vi "Get Image Item Ref.vi"(8 "error in (no error)":errorcluster caption="错误输入（无错误）", 10 "index":i32, 11 "ImageListClass 输入":refnum<class "ImageListClass.lvclass"> caption="DNL_LabVIEW Object in") -> (0 "error out":errorcluster caption="错误输出", 2 "get_Item":refnum<k24>, 3 "ImageListClass 输出":refnum<class "ImageListClass.lvclass"> caption="DNL_LabVIEW Object out")   [LabVIEW 2013, in "ImageListClass.lvclass"]
uses:
  ImageListClass.lvclass
  System.Drawing
  ImageListClass.lvclass/ImageListClass.ctl
  System.Windows.Forms
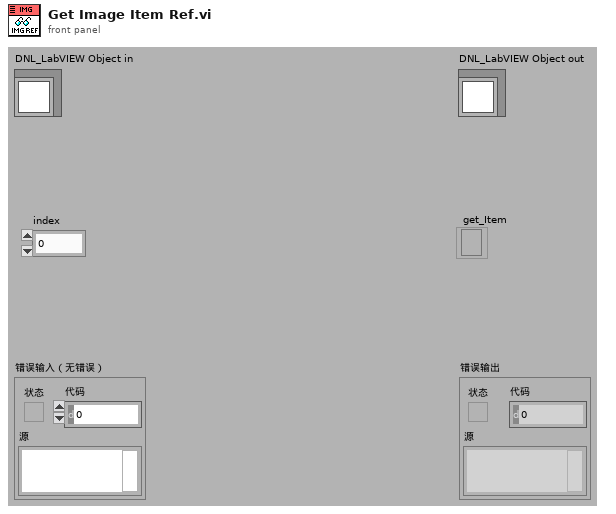
[diagram p1: front panel]
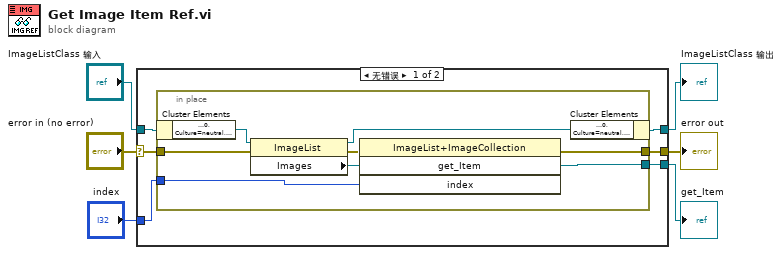
[diagram p0: block diagram]
diagram:
  n1 = case shown="无错误" "error in (no error)" {
    selector: "error in (no error)" -> [w8 w22]
    tunnel: [w7 w22] -> w5
    tunnel: [w11 w21] -> w3
    tunnel: "ImageListClass 输入" -> [w12 w21]
    tunnel: "index" -> [w10 _]
    tunnel: [w9 _] -> w1
    frame No Error {
      n2 = in-place {
        in-place-border: w10 -> [w18]
        in-place-border: [w17] -> w9
        in-place-border: w8 -> [w15]
        in-place-border: [w13] -> w7
        n3 = in-place-cluster #1(w12) -> ("ImageList"=w20:refnum<k24>)
        n4 = property class="ImageList"(reference=w20, error in=w15) -> (reference out=w16:refnum<k24>, error out=w14:errorcluster, "Images"=w19:refnum<k24>)
        n5 = invoke class="ImageList+ImageCollection" method="get_Item"(reference=w19, error in=w14, "index"=w18) -> (error out=w13:errorcluster, "get_Item"=w17:refnum<k24>)  [unwired: 1 in, 2 out]
        n6 = in-place-cluster #1("ImageList"=w16) -> (w11:refnum<class "ImageListClass.lvclass">)
      }
    }
    frame Error {
    }
  }
  "error out" <- w5
  "ImageListClass 输出" <- w3
  "get_Item" <- w1
